vi "Configure Multi Eval Meas Limit ACLR Test Tolerance.vi"(7 "Tolerance 6 GHz (0.0)":dbl format="%^.3e", 8 "error in (no error)":errorcluster, 9 "Tolerance 4 GHz (0.0)":dbl format="%^.3e", 10 "Instance (1)":T1=1, 11 "VISA resource name":refnum<visa-resource-name>) -> (0 "error out":errorcluster, 3 "VISA resource name out":refnum<visa-resource-name>)   [LabVIEW 2020, in "Rohde&Schwarz CMWXP NR FR1 Measurement.lvlib"]
doc: "Defines the test tolerance for relative ACLR limits, depending on the carrier frequency.\n\nAttribute:\nRSCMWXPNRFR1M_ATTR_MULTI_EVAL_MEAS_LIMIT_ACLR_TEST_TOLERANCE\n\nRemote-control command:\nCONFigure:NRSub:MEAS<i>:MEValuation:LIMit:ACLR:TTOLerance"
uses:
  <instrlib>/Rohde&Schwarz CMWXP NR FR1 Measurement/Rohde&Schwarz CMWXP NR FR1 Measurement.lvlib
  <instrlib>/Rohde&Schwarz CMWXP NR FR1 Measurement/Private/_Instance.ctl
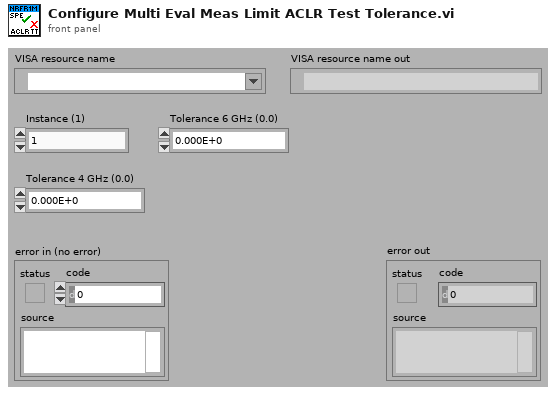
[diagram p1: front panel]
types:
  T1 = typedef "Rohde&Schwarz CMWXP NR FR1 Measurement.lvlib/_Instance.ctl" = i32
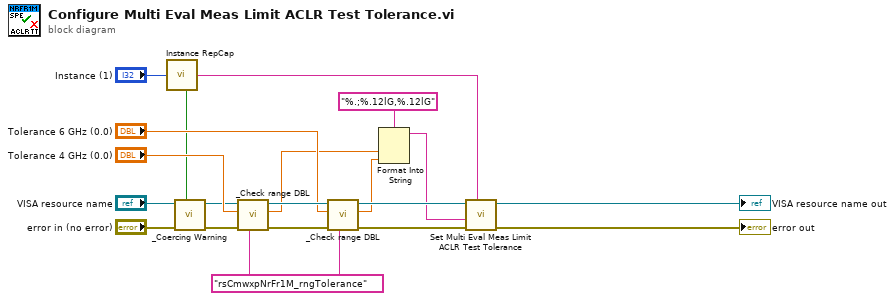
[diagram p0: block diagram]
diagram:
  w12 = "rsCmwxpNrFr1M_rngTolerance" ("Range Table Identifier")
  n1 = call <instrlib>:"Instance RepCap.vi"("Instance In"="Instance (1)") -> ("In Range?"=w1:bool, "RepCap Identifier Out"=w10:string)  [unwired: 1 in]
  n2 = call <instrlib>:"_Coercing Warning.vi"("In Range?"=w1, "error in (no error)"="error in (no error)", "VISA resource name"="VISA resource name") -> ("error out"=w3:errorcluster, "VISA resource name out"=w2:refnum<visa-resource-name>)  [unwired: 7 in]
  n3 = call <instrlib>:"_Check range DBL.vi"("Range Table Identifier"=w12, "error in (no error)"=w3, "DBL Value In"="Tolerance 4 GHz (0.0)", "VISA resource name"=w2) -> ("error out"=w18:errorcluster, "DBL Value Out"=w8:dbl, "VISA resource name out"=w17:refnum<visa-resource-name>)  [unwired: 5 in]
  n4 = call <instrlib>:"_Check range DBL.vi"("Range Table Identifier"=w12, "error in (no error)"=w18, "DBL Value In"="Tolerance 6 GHz (0.0)", "VISA resource name"=w17) -> ("error out"=w16:errorcluster, "DBL Value Out"=w7:dbl, "VISA resource name out"=w15:refnum<visa-resource-name>)  [unwired: 5 in]
  n5 = Format Into String(format string="%.;%.12lG,%.12lG", w8, w7) -> (resulting string=w6:string)  [unwired: 2 in, 1 out]
  n6 = call "Set Multi Eval Meas Limit ACLR Test Tolerance"("Repeated Capabilities"=w10, "error in (no error)"=w16, "Multi Eval Meas Limit ACLR Test Tolerance ()"=w6, "instrument handle"=w15) -> ("error out"=→"error out":errorcluster, "instrument handle out"=→"VISA resource name out":refnum<visa-resource-name>)  [unwired: 6 in]
